vi "RT Main.vi"   [LabVIEW 2014]
types:
  T1 = typedef "Track (File) References.ctl" = cluster{"Track_1_Ref":refnum<k34>, "Track_2_Ref":refnum<k34>, "Track_3_Ref":refnum<k34>, "Track_4_Ref":refnum<k34>, "Track_Name_1":string, "Track_Name_2":string, "Track_Name_3":string, "Track_Name_4":string}
  T2 = typedef "FPGA Reference.ctl" = refnum<k20>
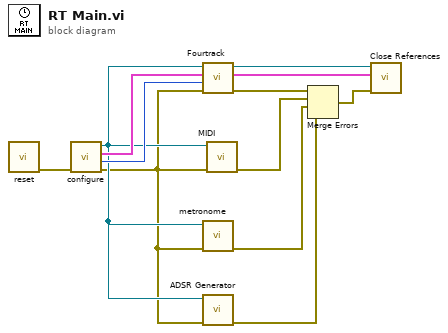
[diagram p0: block diagram]
diagram:
  n1 = call "reset.vi"() -> ("error out"=w7:errorcluster)  [unwired: 11 in]
  n2 = call "configure.vi"("error in (no error)"=w7) -> ("error out"=w3:errorcluster, "Track Division in Samples"=w9:i32, "Track (File) References"=w8:T1, "Refnum Out"=w4:T2)  [unwired: 7 in]
  n3 = call "Fourtrack.vi"("error in (no error)"=w3, "Track Division in Samples"=w9, "Track (File) References in"=w8, "Refnum in"=w4) -> ("error out"=w6:errorcluster, "Track (File) References out"=w11:T1, "Refnum out"=w12:T2)  [unwired: 5 in]
  n4 = call "metronome.vi"("error in (no error)"=w3, "Refnum in"=w4) -> ("error out"=w2:errorcluster)  [unwired: 9 in]
  n5 = call "ADSR Generator.vi"("error in"=w3, "FPGA VI Reference In"=w4) -> ("error out"=w1:errorcluster)  [unwired: 9 in]
  n6 = call "MIDI.vi"("error in (no error)"=w3, "Refnum in"=w4) -> ("error out"=w10:errorcluster)  [unwired: 9 in]
  n7 = Merge Errors(w6, w10, w2, w1) -> (w5:errorcluster)
  n8 = call "Close References.vi"("error in (no error)"=w5, "Track (File) References"=w11, "Refnum in"=w12) -> ()  [unwired: 9 in]
